vi "st_Poisson Inverse CDF (kx).vi"(10 "lambda":dbl=1.0, 11 "cdf(x)":dbl=0.999) -> (0 "error":i32, 3 "x":dbl=4.722291756604139)   [LabVIEW 2020, in "NI_Gmath.lvlib"]
uses:
  <vilib>/gmath/NI_Gmath.lvlib
  <vilib>/gmath/statdist.llb/st_error_code.ctl
panel:
  # "Poisson Inverse CDF"
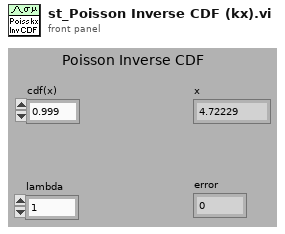
[diagram p1: front panel]
types:
  T1 = typedef "NI_Gmath.lvlib/st_error_code.ctl" = i32
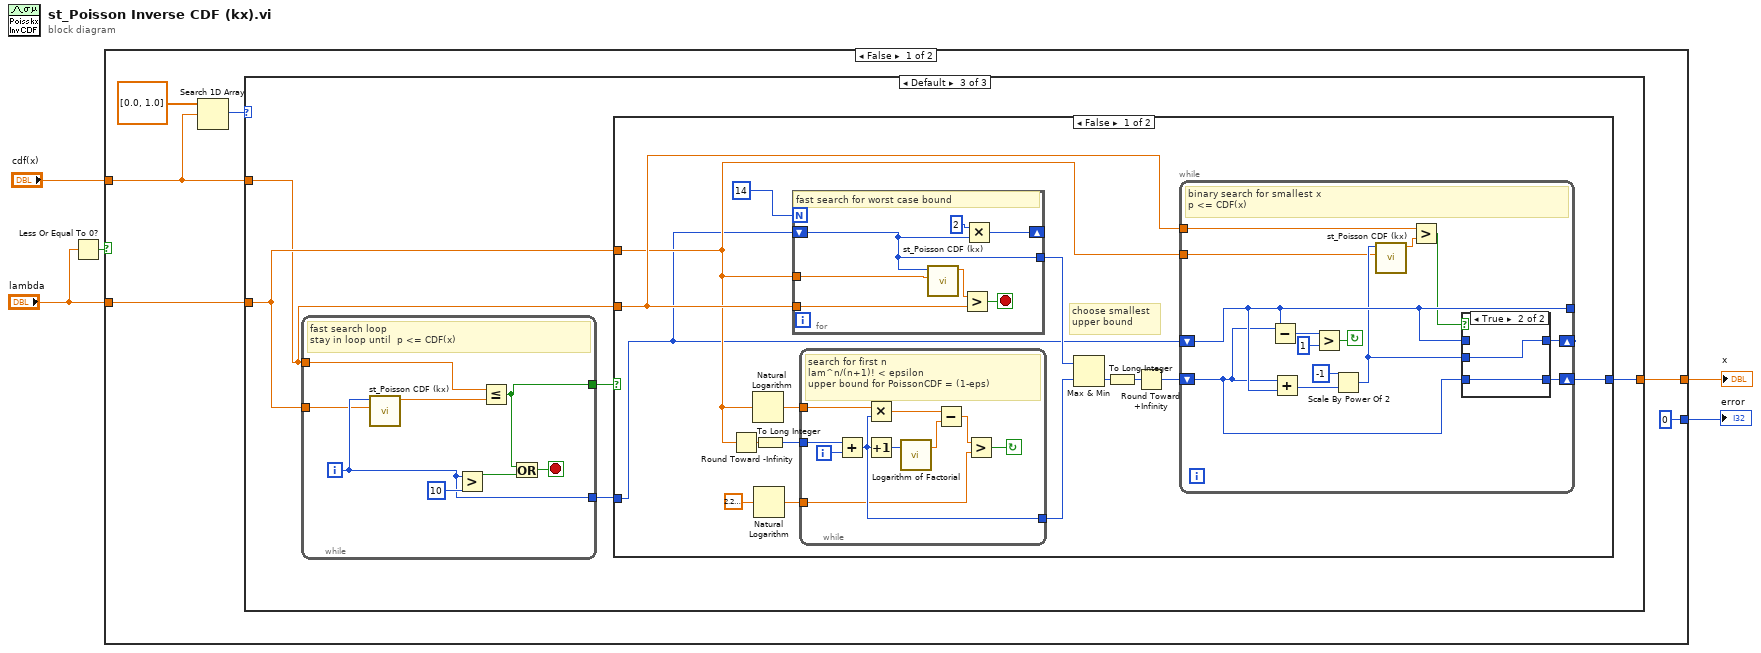
[diagram p0: block diagram]
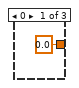
[diagram p2: hidden frame]
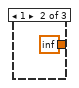
[diagram p3: hidden frame]
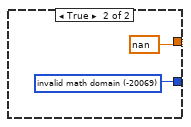
[diagram p6: hidden frame]
diagram:
  n1 = Less Or Equal To 0?(x="lambda") -> (x <= 0?=w1:bool)
  n2 = case shown="False" w1 {
    tunnel: "lambda" -> [w9 _]
    tunnel: [0 ("invalid math domain") w78] -> w5
    tunnel: [w10 nan] -> w4
    tunnel: "cdf(x)" -> [w6 _]
    frame False {
      n3 = Search 1D Array(1D array=dbl[] [0.0, 1.0], element=w6) -> (index of element=w7:i32)  [unwired: 1 in]
      n4 = case shown="Default" w7 {
        tunnel: [0.0 ("zero") inf ("zero") w14] -> w10
        tunnel: w6 -> [_ _ w15]
        tunnel: w9 -> [_ _ w16]
        frame 0 {
        }
        frame 1 {
        }
        frame Default {
          n5 = while {
            tunnel: w16 -> [w70]
            tunnel: w15 -> [w74]
            tunnel: [w73] -> w18
            tunnel: [w71] -> w17
            i -> [w71]
            stop <- w75 stop-if-true
            # "fast search loop\nstay in loop until  p <= CDF(x)"
            n6 = call <vilib>:"st_Poisson CDF (kx).vi"("a"=w70, "x"=w71) -> ("cdf(x)"=w72:dbl)  [unwired: 8 in, 1 out]
            n7 = Greater?(x=w71, y=10) -> (0:w76:bool)
            n8 = Less Or Equal?(x=w74, y=w72) -> (x <= y?=w73:bool)
            n9 = Or(x=w73, y=w76) -> (x .or. y?=w75:bool)
          }
          n10 = case shown="False" w18 {
            tunnel: w15 -> [w23 _]
            tunnel: w16 -> [w21 _]
            tunnel: [w20 w69] -> w14
            tunnel: w17 -> [w19 w69]
            frame False {
              # "choose smallest \nupper bound"
              n11 = Round Toward -Infinity(1:w21) -> (0:w32:dbl)
              n12 = Natural Logarithm(1:w21) -> (0:w28:dbl)
              n13 = Natural Logarithm(1:2.220446049250313e-16) -> (0:w29:dbl)
              n14 = To Long Integer(number=w32) -> (32bit integer=w31:i32)
              n15 = for {
                N: 14 -> [_]
                shift-right: [w67] -> _
                shift-left: w19 -> [w62]
                tunnel: w21 -> [w66]
                tunnel: w23 -> [w64]
                tunnel: [w62] -> w27
                stop <- w63 stop-if-true
                # "fast search for worst case bound"
                n16 = call <vilib>:"st_Poisson CDF (kx).vi"("a"=w66, "x"=w62) -> ("cdf(x)"=w65:dbl)  [unwired: 8 in, 1 out]
                n17 = Greater?(x=w65, y=w64) -> (0:w63:bool)
                n18 = Multiply(x=2, y=w62) -> (x*y=w67:i32)
              }
              n19 = while {
                tunnel: w31 -> [w56]
                tunnel: [w54] -> w26
                tunnel: w29 -> [w53]
                tunnel: w28 -> [w52]
                i -> [w55]
                stop <- w57 continue-if-true
                # "search for first n\nlam^n/(n+1)! < epsilon\nupper bound for PoissonCDF = (1-eps)"
                n20 = Add(x=w56, y=w55) -> (x+y=w54:i32)
                n21 = Multiply(x=w52, y=w54) -> (x*y=w59:dbl)
                n22 = Increment(x=w54) -> (x+1=w61:i32)
                n23 = call <vilib>:"Logarithm of Factorial.vi"("n"=w61) -> ("ln(n!)"=w60:dbl)  [unwired: 2 in]
                n24 = Subtract(x=w59, y=w60) -> (x-y=w58:dbl)
                n25 = Greater?(x=w58, y=w53) -> (0:w57:bool)
              }
              n26 = Max & Min(x=w27, y=w26) -> (min(x,y)=w25:i32)  [unwired: 1 out]
              n27 = Round Toward +Infinity(x=w25) -> (ceil(x): smallest int >= x=w24:i32)
              n28 = To Long Integer(number=w24) -> (32bit integer=w22:i32)
              n29 = while {
                shift-right: [w41] -> _
                shift-left: w19 -> [w39]
                shift-right: [w40] -> w20
                shift-left: w22 -> [w38]
                tunnel: [w39] -> _
                tunnel: w23 -> [w42]
                tunnel: w21 -> [w36]
                stop <- w45 continue-if-true
                # "binary search for smallest x\np <= CDF(x)"
                n30 = Subtract(x=w38, y=w39) -> (x-y=w47:i32)
                n31 = Add(x=w38, y=w39) -> (x+y=w44:i32)
                n32 = Greater?(x=w47, y=1) -> (0:w45:bool)
                n33 = Scale By Power Of 2(n=-1, x=w44) -> (x*2^n=w37:i32)
                n34 = call <vilib>:"st_Poisson CDF (kx).vi"("a"=w36, "x"=w37) -> ("cdf(x)"=w35:dbl)  [unwired: 8 in, 1 out]
                n35 = Greater?(x=w42, y=w35) -> (0:w34:bool)
                n36 = case shown="True" w34 {
                  tunnel: w37 -> [w49 w51]
                  tunnel: [w48 w51] -> w41
                  tunnel: [w49 w50] -> w40
                  tunnel: w38 -> [_ w50]
                  tunnel: w39 -> [w48 _]
                  frame False {
                  }
                  frame True {
                  }
                }
              }
            }
            frame True {
            }
          }
        }
      }
    }
    frame True {
      w78 = T1 -20069 items=["invalid math domain"=-20069, "Fourier interpolation size m >= n"=-20070, "empty array"=-20003] ("stat interp error code")
    }
  }
  "x" <- w4
  "error" <- w5
